vi "Section07_UpdateUI-05-UpdateStatusString.vi"(8 "error in (no error)":errorcluster, 10 "Variant Data":variant, 11 "QSM_ShiftRegister_UpdateUI_In in":T1) -> (0 "error out":errorcluster, 3 "QSM_ShiftRegister_UpdateUI_In out":T1)   [LabVIEW 2014, in "GUIUpdateQSM.lvlib"]
uses:
  GUIUpdateQSM.lvlib
  Controls/QSM_ShiftRegister.ctl
  QueueMaintenance/TypeDef/QSMRef_ALL.ctl
  Controls/QSM_Reference.ctl
  Controls/QSM_DataType.ctl
  Controls/QSM_RunStates.ctl
  Queue_TEST/Controls/QSM_Reference.ctl
  Queue_TEST/Controls/QSM_DataType.ctl
  Queue_TEST/Controls/QSM_RunStates.ctl
  Controls/TypeDef_FrontPanelReferences.ctl
  QueueMaintenance/QueueMaintenance.lvlib
  Queue_TEST/TestQSM.lvlib
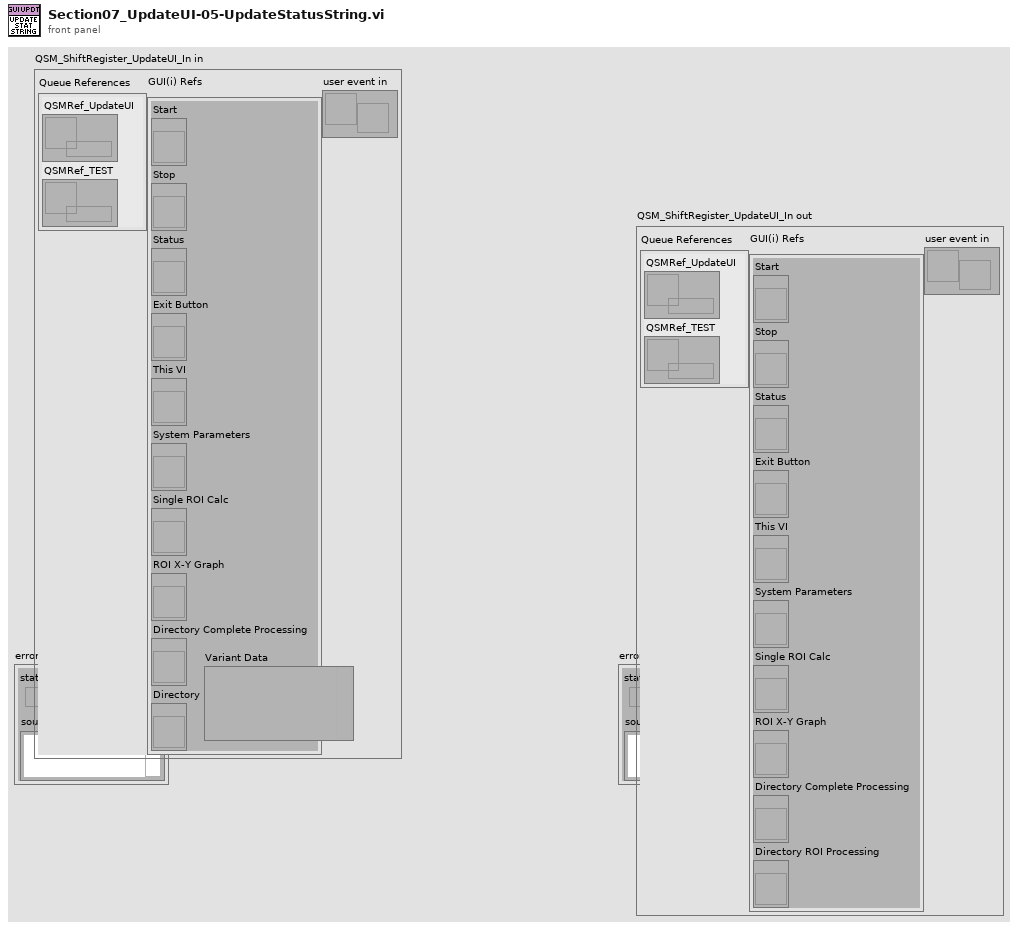
[diagram p1: front panel]
types:
  T1 = typedef "GUIUpdateQSM.lvlib/QSM_ShiftRegister.ctl" = cluster{"Queue References":T2, "GUI(i) Refs":T5, "user event in":refnum<user-event>}
  T2 = typedef "QueueMaintenance.lvlib/QSMRef_ALL.ctl" = cluster{"QSMRef_UpdateUI":T3, "QSMRef_TEST":T4}
  T3 = typedef "GUIUpdateQSM.lvlib/QSM_Reference.ctl" = refnum<queue>
  T4 = typedef "TestQSM.lvlib/QSM_Reference.ctl" = refnum<queue>
  T5 = typedef "GUIUpdateQSM.lvlib/TypeDef_FrontPanelReferences.ctl" = cluster{"Start":refnum<vi>, "Stop":refnum<vi>, "Status":refnum<vi>, "Exit Button":refnum<vi>, "This VI":refnum<vi>, "System Parameters":refnum<vi>, "Single ROI Calc":refnum<vi>, "ROI X-Y Graph":refnum<vi>, "Directory Complete Processing":refnum<vi>, "Directory ROI Processing":refnum<vi>}
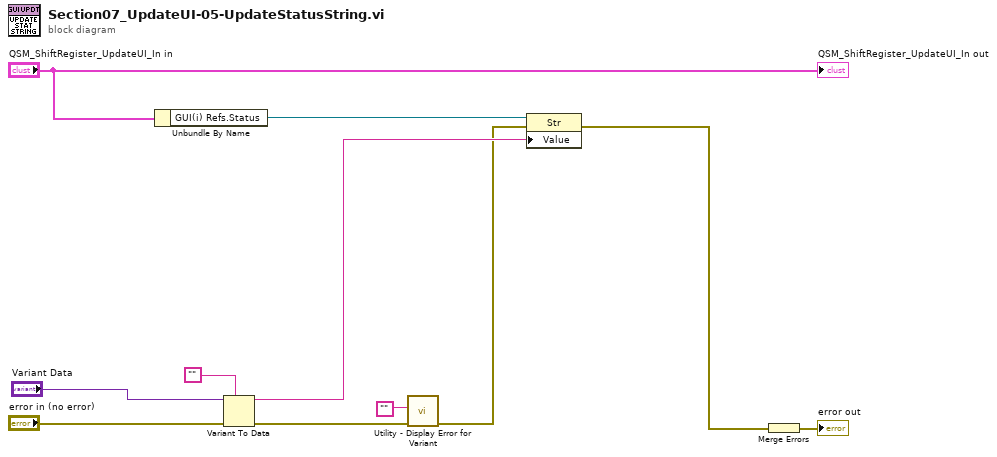
[diagram p0: block diagram]
diagram:
  n1 = Unbundle By Name("QSM_ShiftRegister_UpdateUI_In in") -> ("GUI(i) Refs.Status"=w10:refnum<vi>)
  n2 = Variant To Data(error in="error in (no error)", type="", Variant="Variant Data") -> (data=w4:string, error out=w3:errorcluster)
  n3 = call "Utility - Display Error for Variant.vi"("error in (no error)"=w3, "Step"="") -> ("error out"=w2:errorcluster)  [unwired: 9 in]
  n4 = property class="Str"(reference=w10, error in=w2, "Value"=w4) -> (error out=w9:errorcluster)  [unwired: 1 out]
  n5 = Merge Errors(w9) -> (→"error out":errorcluster)
  "QSM_ShiftRegister_UpdateUI_In out" <- "QSM_ShiftRegister_UpdateUI_In in"
